vi "EXDIR-YAML_IsFloatingColonLine.vi"(11 "Line":string) -> (3 "line ends with floating colon":bool)   [LabVIEW 2016]
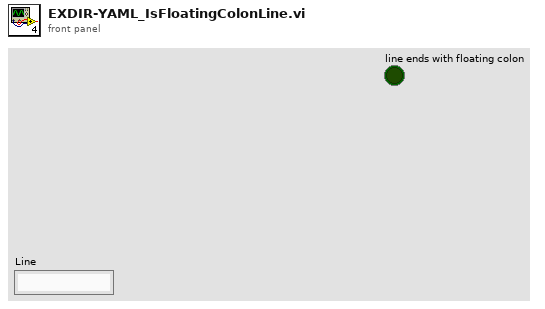
[diagram p1: front panel]
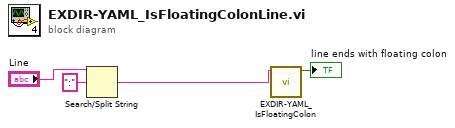
[diagram p0: block diagram]
diagram:
  n1 = Search/Split String(string="Line", search string/char (-)=":") -> (match + rest of string=w2:string)  [unwired: 1 in, 2 out]
  n2 = call "EXDIR-YAML_IsFloatingColon.vi"("String"=w2) -> ("after the 1st char is empty or all spaces"=→"line ends with floating colon":bool)  [unwired: 10 in]
